vi "air_flow_video.vi"() -> ()   [LabVIEW 2020]
uses:
  <vilib>/ptbypt/NI_PtbyPt.lvlib
panel:
  out "Error":bool
  out "time string":string
  out "x-y":dbl
  out "output":i32
  in  "stop":bool
  out "Waveform Chart":cluster{i32, "median":dbl}(graph)
  out "Output string":string
  out "Image":T1(plugin-control)
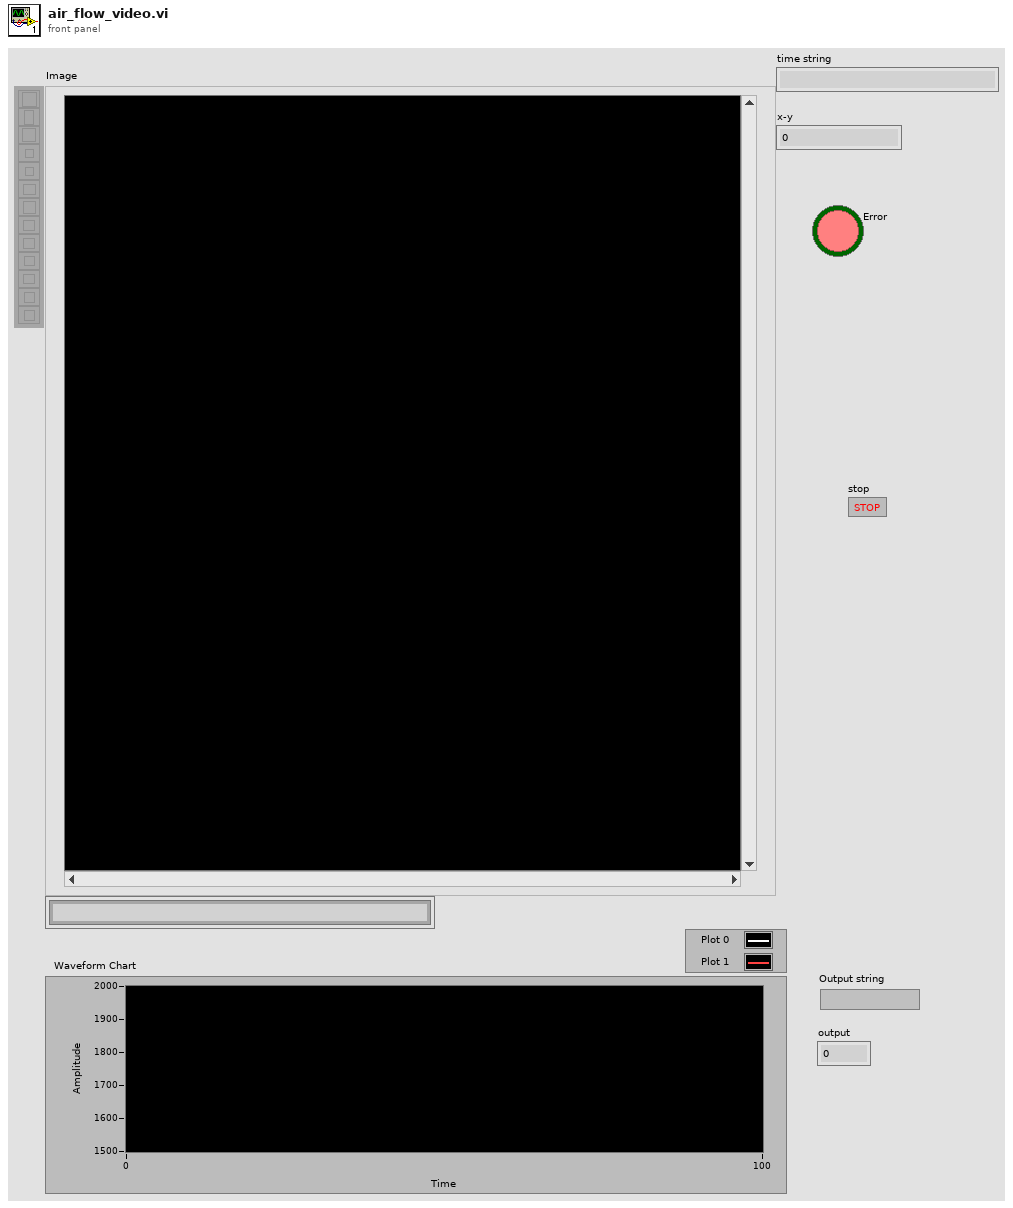
[diagram p1: front panel]
types:
  T1 = typedef "IMAQ Image.ctl" = refnum<image>
  T2 = typedef "Image Type" = u32
  T3 = typedef "IMAQ AVI2 Refnum.ctl" = refnum<k20>
  T4 = cluster{"Left":i32, "Top":i32, "Right":i32, "Bottom":i32}
  T5 = cluster{"Global Rectangle":i32[], "Contours":cluster{"ID":enum32{"External", "Internal"}, "Type":u32, "Coordinates":i32[]}[]}
  T6 = typedef "IMAQ Rectangle" = cluster{"Left":i32, "Top":i32, "Right":i32, "Bottom":i32, "Rotation":dbl}
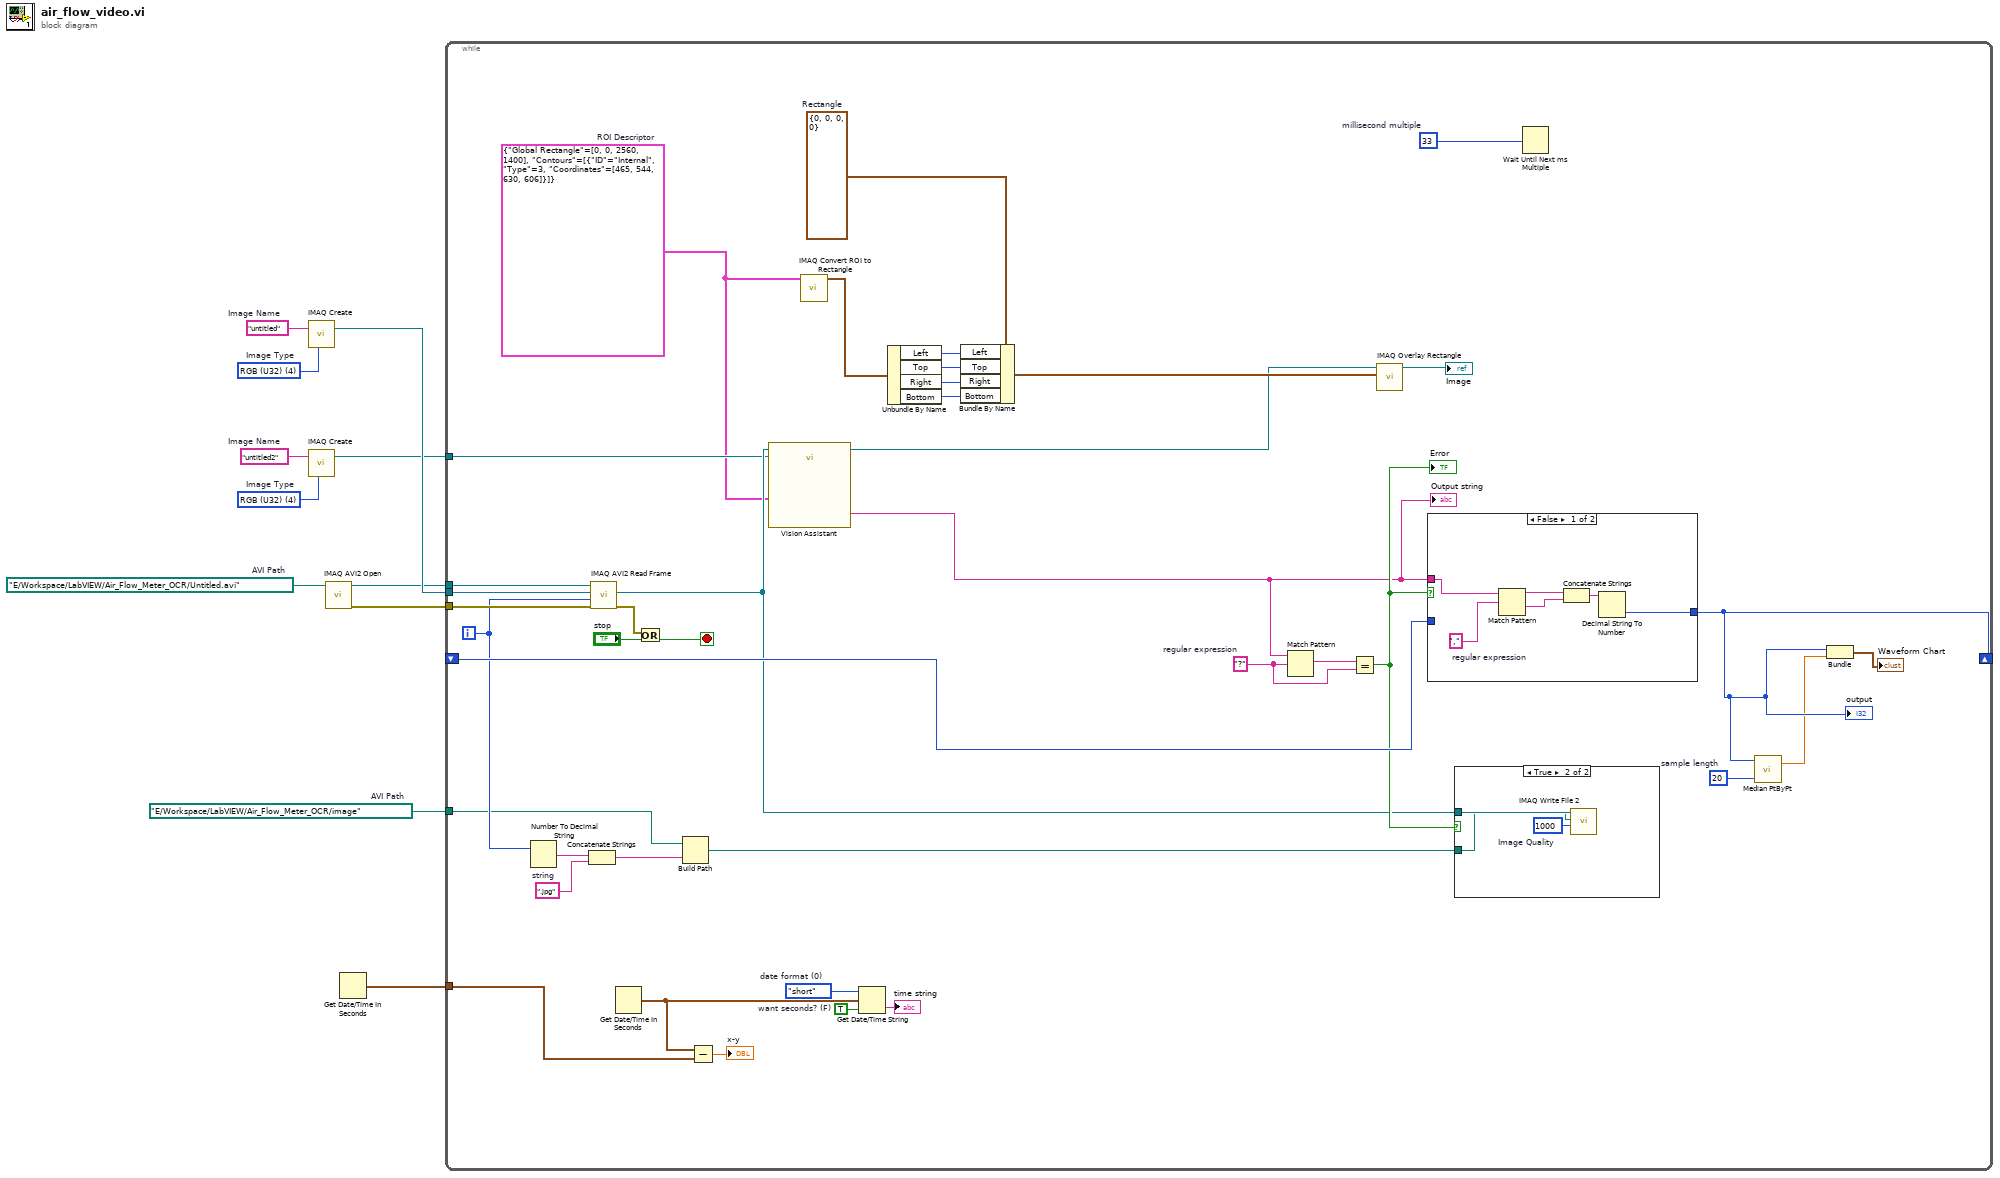
[diagram p0: block diagram]
diagram:
  w1 = path "E:/Workspace/LabVIEW/Air_Flow_Meter_OCR/image"  # AVI Path
  w5 = T2 4 items=["Grayscale (U8)", "Grayscale (I16)", "Grayscale (SGL)", "Complex (CSG)", "RGB (U32)", "HSL (U32)", "RGB (U64)", "Grayscale (U16)"]  # Image Type
  w4 = "untitled2"  # Image Name
  w8 = path "E:/Workspace/LabVIEW/Air_Flow_Meter_OCR/Untitled.avi"  # AVI Path
  w10 = T2 4 items=["Grayscale (U8)", "Grayscale (I16)", "Grayscale (SGL)", "Complex (CSG)", "RGB (U32)", "HSL (U32)", "RGB (U64)", "Grayscale (U16)"]  # Image Type
  w11 = "untitled"  # Image Name
  n1 = call "IMAQ Create"("Image Name"=w11, "Image Type"=w10) -> ("New Image"=w9:T1)  [unwired: 3 in, 1 out]
  n2 = call "IMAQ Create"("Image Name"=w4, "Image Type"=w5) -> ("New Image"=w3:T1)  [unwired: 3 in, 1 out]
  n3 = call "IMAQ AVI2 Open"("AVI File Path"=w8) -> ("error out"=w6:errorcluster, "AVI Refnum"=w7:T3)  [unwired: 9 in]
  n4 = Get Date/Time In Seconds() -> (seconds since 1Jan1904=w2:timestamp)
  n5 = while {
    tunnel: w7 -> [w43]
    tunnel: w9 -> [w42]
    tunnel: w6 -> [w39]
    tunnel: w3 -> [w19]
    shift-right: [w14] -> _
    shift-left: _ -> [w36]
    tunnel: w2 -> [w35]
    tunnel: w1 -> [w23]
    i -> [w25]
    stop <- w29 stop-if-true
    w15 = 20  # sample length
    w21 = ".jpg"  # string
    w30 = enum16{"short", "long", "abbreviated"}."short"  # date format (0)
    w31 = TRUE  # want seconds? (F)
    w37 = "?"  # regular expression
    w41 = u32 33  # millisecond multiple
    w50 = T4 {"Left"=0, "Top"=0, "Right"=0, "Bottom"=0}  # Rectangle
    w18 = T5 {"Global Rectangle"=[0, 0, 2560, 1400], "Contours"=[{"ID"=enum."Internal", "Type"=3, "Coordinates"=[465, 544, 630, 606]}]}  # ROI Descriptor
    n6 = Number To Decimal String(number=w25) -> (decimal integer string=w24:string)  [unwired: 1 in]
    n7 = Concatenate Strings(w24, w21) -> (w22:string)
    n8 = call "IMAQ AVI2 Read Frame"("error in (no error)"=w39, "Frame Number"=w25, "Image"=w42, "AVI Refnum"=w43) -> ("error out"=w28:errorcluster, "Image Out"=w20:T1)  [unwired: 5 in, 1 out]
    n9 = Get Date/Time In Seconds() -> (seconds since 1Jan1904=w33:timestamp)
    n10 = Or(x=w28, y="stop") -> (x .or. y?=w29:bool)
    n11 = Build Path(base path=w23, name or relative path=w22) -> (appended path=w26:path)
    n12 = Subtract(x=w33, y=w35) -> (x-y=→"x-y":dbl)
    n13 = call "Vision Assistant"("Image In"=w20, "Image Dst"=w19, "ROI Descriptor (OCR/OCV 1)"=w18) -> ("Image Out"=w17:T1, "String (OCR/OCV 1)"=w16:string)  [unwired: 22 in, 1 out]
    "Output string" <- w16
    n14 = call "IMAQ Convert ROI to Rectangle"("ROI Descriptor"=w18) -> ("Rectangle"=w51:T6)  [unwired: 8 in, 1 out]
    n15 = Get Date/Time String(date format (0)=w30, seconds (now)=w33, want seconds? (F)=w31) -> (time string=→"time string":string)  [unwired: 1 out]
    n16 = Unbundle By Name(w51) -> ("Left"=w49:i32, "Top"=w48:i32, "Right"=w47:i32, "Bottom"=w46:i32)
    n17 = Bundle By Name(cluster=w50, "Left"=w49, "Top"=w48, "Right"=w47, "Bottom"=w46) -> (w45:T4)
    n18 = Match Pattern(string=w16, regular expression=w37) -> (match substring=w38:string)  [unwired: 1 in, 3 out]
    n19 = Equal?(x=w38, y=w37) -> (x = y?=w27:bool)
    "Error" <- w27
    n20 = call "IMAQ Overlay Rectangle"("Rectangle"=w45, "Image"=w17) -> ("Image Out"=→"Image":T1)  [unwired: 8 in, 1 out]
    n21 = case shown="False" w27 {
      tunnel: [w56 w61] -> w14
      tunnel: w16 -> [w55 _]
      tunnel: w36 -> [_ w61]
      frame False {
        w60 = ","  # regular expression
        n22 = Match Pattern(string=w55, regular expression=w60) -> (before substring=w59:string, after substring=w58:string)  [unwired: 1 in, 2 out]
        n23 = Concatenate Strings(w59, w58) -> (w57:string)
        n24 = Decimal String To Number(string=w57) -> (number=w56:i32)  [unwired: 2 in, 1 out]
      }
      frame True {
      }
    }
    "output" <- w14
    n25 = case shown="True" w27 {
      tunnel: w20 -> [_ w54]
      tunnel: w26 -> [_ w52]
      frame False {
      }
      frame True {
        w53 = u32 1000  # Image Quality
        n26 = call-poly "IMAQ Write File 2"("Image Quality"=w53, "File Path"=w52, "Image"=w54) -> ()  [unwired: 7 in, 2 out]
      }
    }
    n27 = Wait Until Next ms Multiple(millisecond multiple=w41) -> ()  [unwired: 1 out]
    n28 = call <vilib>:"Median PtByPt.vi"("sample length"=w15, "x"=w14) -> ("median"=w13:dbl)  [unwired: 2 in, 1 out]
    n29 = Bundle(w14, "median"=w13) -> (→"Waveform Chart":cluster{i32, "median":dbl})  [unwired: 1 in]
  }
